vi "Get stack data.vi"(8 "error in (no error)":errorcluster, 10 "Last Index for Type":dbl, 11 "Stack in":refnum<class "Stack.lvclass">) -> (0 "error out":errorcluster, 2 "Data cluster":T1={"type"="proto", " geometry"="full", "resolution"="LD", "baselayer"="BA_123", "toplayer"="SI_789", "bl_pos"="1", "tl_pos"="1", "put_pos"="1", "region"="1", "asstray"="1", "comptray"="1", "put"="1", "date"="2024-04-02", "timestart"="1:12:12.442", "timeend"="1:23:45.244", "operator"="cmuperson", "tape"="some", "glue"="some", "stack name"="some"}, 3 "Stack out":refnum<class "Stack.lvclass">)   [LabVIEW 2021, in "Stack.lvclass"]
uses:
  Stack.lvclass
  Stack.lvclass/Stack.ctl
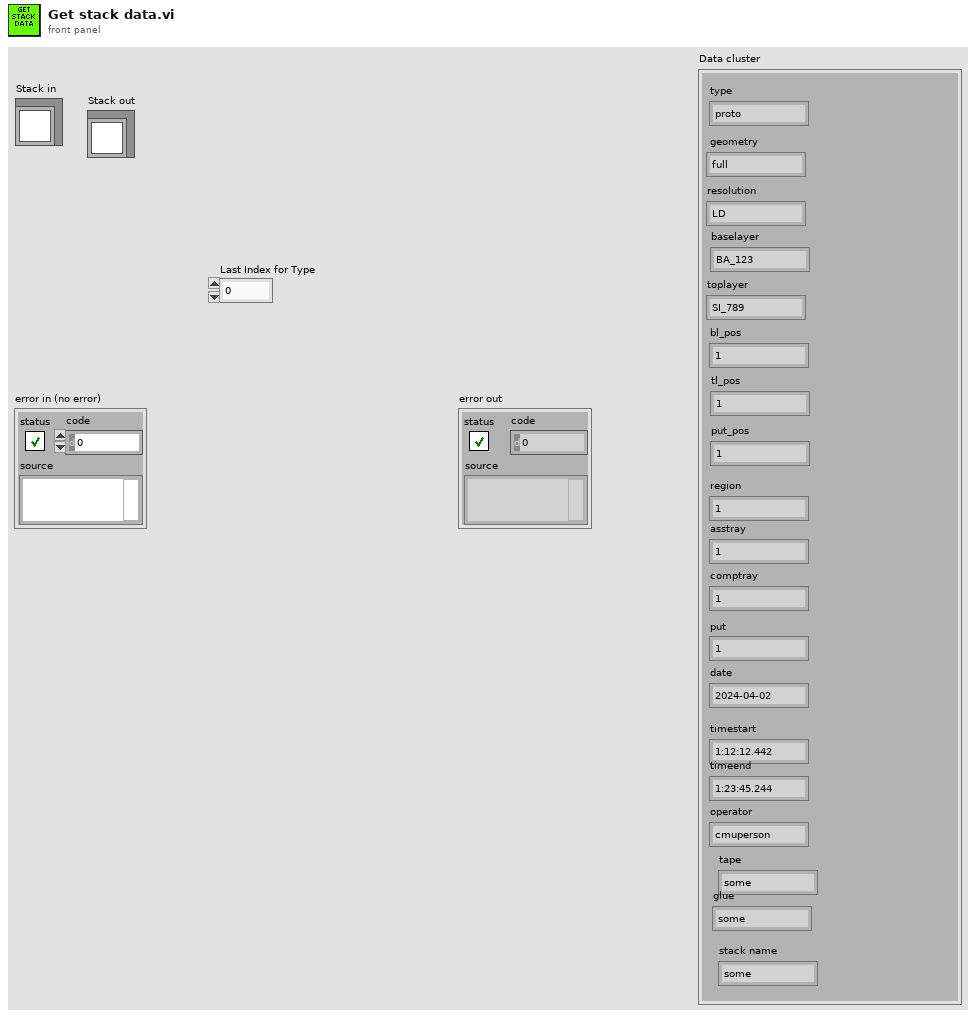
[diagram p1: front panel]
types:
  T1 = cluster{"type":string, " geometry":string, "resolution":string, "baselayer":string, "toplayer":string, "bl_pos":string, "tl_pos":string, "put_pos":string, "region":string, "asstray":string, "comptray":string, "put":string, "date":string, "timestart":string, "timeend":string, "operator":string, "tape":string, "glue":string, "stack name":string}
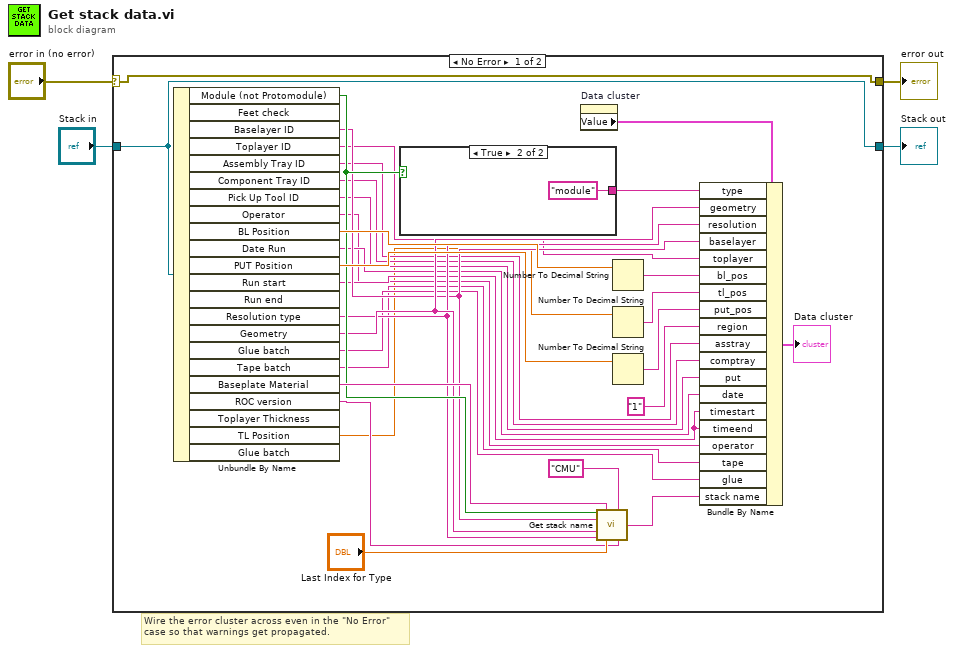
[diagram p0: block diagram]
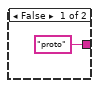
[diagram p2: hidden frame]
diagram:
  # "Wire the error cluster across even in the \"No Error\"\ncase so that warnings get propagated."
  n1 = case shown="No Error" "error in (no error)" {
    selector: "error in (no error)" -> [w34 w38]
    tunnel: [w34 w38] -> w3
    tunnel: [w33 w37] -> w1
    tunnel: "Stack in" -> [w33 w37]
    frame No Error {
      n2 = Unbundle By Name(w33) -> ("Module (not Protomodule)"=w28:bool, "Baselayer ID"=w19:string, "Toplayer ID"=w18:string, "Assembly Tray ID"=w17:string, "Component Tray ID"=w16:string, "Pick Up Tool ID"=w15:string, "Operator"=w12:string, "BL Position"=w32:dbl, "Date Run"=w14:string, "PUT Position"=w31:dbl, "Run start"=w13:string, "Resolution type"=w20:string, "Geometry"=w21:string, "Glue batch"=w11:string, "Tape batch"=w10:string, "Baseplate Material"=w29:string, "ROC version"=w26:string, "TL Position"=w9:dbl)  [unwired: 4 out]
      n3 = case shown="True" w28 {
        tunnel: ["proto" ("type") "module" ("type")] -> w22
        frame False {
        }
        frame True {
        }
      }
      n4 = property on="Data cluster" class="Clust (strict)"() -> ("Value"=w24:T1)  [unwired: 2 in, 2 out]
      n5 = call "Get stack name.vi"("Module?"=w28, "Baseplate Type"=w29, "Institution"="CMU", "Protoname (baselayer)"=w19, "Geometry"=w21, "Resolution"=w20, "Numeric"="Last Index for Type", "Hexaboard ROC version"=w26) -> ("Stack name"=w23:string)  [unwired: 7 in]
      n6 = Number To Decimal String(number=w32) -> (decimal integer string=w7:string)  [unwired: 1 in]
      n7 = Number To Decimal String(number=w9) -> (decimal integer string=w8:string)  [unwired: 1 in]
      n8 = Number To Decimal String(number=w31) -> (decimal integer string=w6:string)  [unwired: 1 in]
      n9 = Bundle By Name(cluster=w24, "type"=w22, "geometry"=w21, "resolution"=w20, "baselayer"=w19, "toplayer"=w18, "bl_pos"=w7, "tl_pos"=w8, "put_pos"=w6, "region"="1", "asstray"=w17, "comptray"=w16, "put"=w15, "date"=w14, "timestart"=w13, "timeend"=w13, "operator"=w12, "tape"=w10, "glue"=w11, "stack name"=w23) -> (→"Data cluster":T1)
    }
    frame Error {
    }
  }
  "error out" <- w3
  "Stack out" <- w1
